vi "EVT Camera Set Enum Param.vi"(9 "buffer":string, 10 "name":string, 11 "camera":u64) -> (3 "function return":u32(ring))   [LabVIEW 2019, in "EmergentCameraC.lvlib"]
doc: "EMERGENTCAMERAC_API EVT_ERROR EVT_CameraSetEnumParam(Camera_Handle camera, const char* name, const char* buffer);"
uses:
  EmergentCameraC.lvlib
  emergentInstall_Windows/win64/eSDK/bin/EmergentCameraC.dll
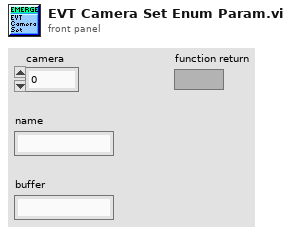
[diagram p1: front panel]
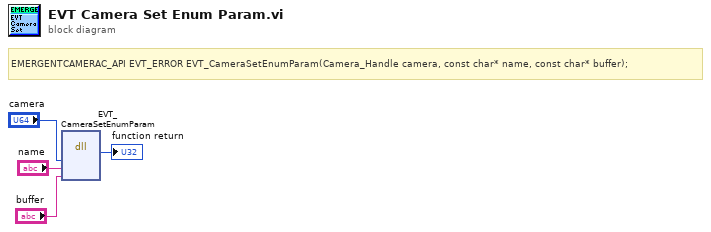
[diagram p0: block diagram]
diagram:
  # "EMERGENTCAMERAC_API EVT_ERROR EVT_CameraSetEnumParam(Camera_Handle camera, const char* name, const char* buffer);"
  n1 = dll-call lib="E:/emergent/host-new_QT/emergentInstall_Windows/win64/eSDK/bin/EmergentCameraC.*" fn="EVT_CameraSetEnumParam"("camera"="camera", "name"="name", "buffer"="buffer") -> (→"function return":u32)  [unwired: 6 in, 2 out]
